vi "Write Value Core.vi"(6 "Owning Write":bool=TRUE, 8 "Name":string, 9 "Existing":bool, 10 "Field Value":T1, 11 "Field ID":T4) -> (2 "Field Value Out":T1)   [LabVIEW 2017]
doc: "Write the value to the variable storage table, notifiy other clients, and update statistics. Doesn't deal with named values, but with IDs."
uses:
  <vilib>/Rock Robotics/Network Tables/Field Data.ctl
  <vilib>/Rock Robotics/Network Tables/Field Type.ctl
  <vilib>/Rock Robotics/Network Tables/Sequence.ctl
  <vilib>/Rock Robotics/Network Tables/Field ID.ctl
  <vilib>/Rock Robotics/Network Tables/NT Globals.vi
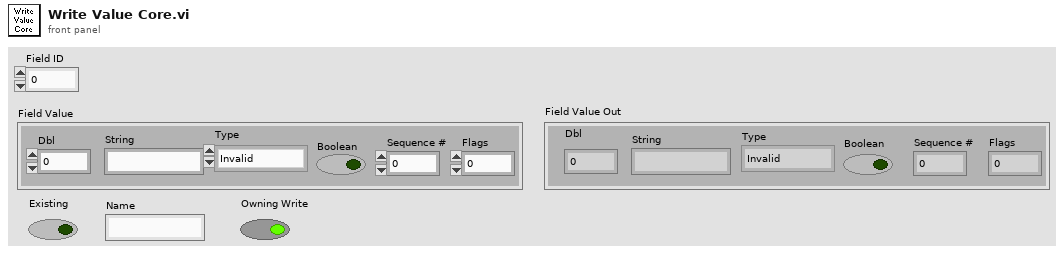
[diagram p1: front panel]
types:
  T1 = typedef "Field Data.ctl" = cluster{"Dbl":dbl, "String":string, "Type":T2, "Boolean":bool, "Sequence #":T3, "Flags":u8}
  T2 = typedef "Field Type.ctl" = enum8{"Invalid", "Bool", "Numeric", "String", "Raw", "Boolean Array", "Numeric Array", "String Array", "RPC"}
  T3 = typedef "Sequence.ctl" = u16
  T4 = typedef "Field ID.ctl" = i32
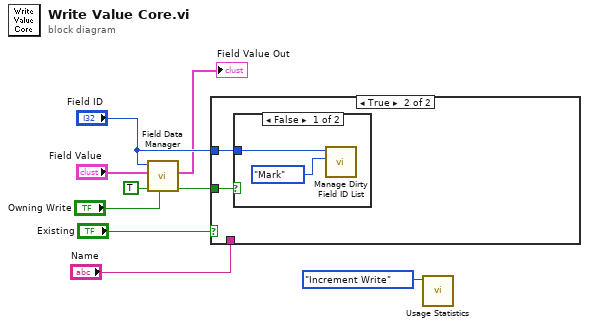
[diagram p0: block diagram]
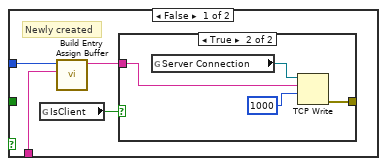
[diagram p2: hidden frame]
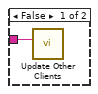
[diagram p3: hidden frame]
diagram:
  n1 = call <vilib>:"Field Data Manager.vi"("Owning Write"="Owning Write", "Increment Sequence"=TRUE, "Field Value In"="Field Value", "Field ID"="Field ID") -> ("Equal"=w8:bool, "Field Value Out"=→"Field Value Out":T1)  [unwired: 6 in]
  n2 = case shown="True" "Existing" {
    tunnel: "Field ID" -> [w13 w20]
    tunnel: w8 -> [_ w19]
    tunnel: "Name" -> [w10 _]
    frame False {
      # "Newly created"
      n3 = global read "NT Globals.vi" "IsClient"() -> (w12:bool)
      n4 = call <vilib>:"Build Entry Assign Buffer.vi"("Name"=w10, "Field ID"=w13) -> ("data string"=w11:string)  [unwired: 9 in]
      n5 = case shown="True" w12 {
        tunnel: w11 -> [w14 w17]
        tunnel: [_ w15] -> _
        frame False {
          n6 = call <vilib>:"Update Other Clients.vi"("data string"=w14) -> ()  [unwired: 11 in]
        }
        frame True {
          n7 = global read "NT Globals.vi" "Server Connection"() -> (w18:refnum<k5>)
          n8 = TCP Write(connection ID=w18, data in=w17, 9:1000 ("timeout ms (25000)")) -> (error out=w15:errorcluster)  [unwired: 1 in, 2 out]
        }
      }
    }
    frame True {
      n9 = case shown="False" w19 {
        tunnel: w20 -> [w22 _]
        frame False {
          n10 = call <vilib>:"Manage Dirty Field ID List.vi"("Operation"=enum16{"Mark", "Retrieve/Clear"}."Mark", "Field ID"=w22) -> ()  [unwired: 8 in, 2 out]
        }
        frame True {
        }
      }
    }
  }
  n11 = call <vilib>:"Usage Statistics.vi"("Operation"=enum16{"Increment Read", "Increment Write"}."Increment Write") -> ()  [unwired: 11 in]
